vi "Shutdown.vi"(8 "error in":errorcluster, 11 "Serial Master in":refnum<class "Serial Master.lvclass">) -> (0 "error out":errorcluster)   [LabVIEW 2021, in "Serial Master.lvclass"]
doc: "This provides an interface for the master to close a connection to the slave."
uses:
  Serial Master.lvclass
  D:/my_projects/projects/Algorithms/Labview/21/Modbus_v121c/Network Protocol/Network Master/Network Master.lvclass
  Network Master.lvclass/Network Master.ctl
  Transmission Data Unit/Transmission Data Unit.lvclass
  Network Master.lvclass
  Serial Master.lvclass/Serial Master.ctl
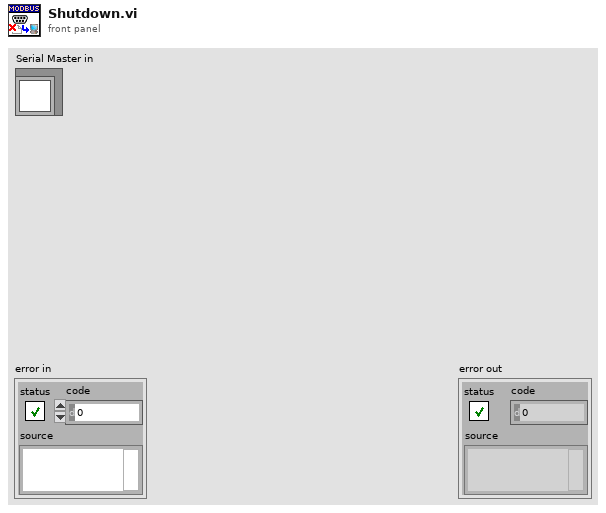
[diagram p1: front panel]
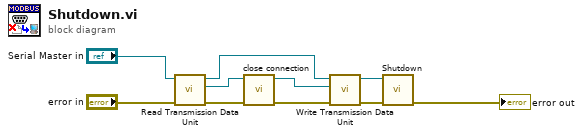
[diagram p0: block diagram]
diagram:
  n1 = call "Read Transmission Data Unit.vi"("error in (no error)"="error in", "Network Master in"="Serial Master in") -> ("error out"=w3:errorcluster, "Transmission Data Unit"=w4:refnum<class "Transmission Data Unit.lvclass">, "Network Master out"=w7:refnum<class "Serial Master.lvclass">)  [unwired: 7 in]
  n2 = call-dynamic "close connection.vi"("error in"=w3, "transmission data unit in"=w4) -> ("error out"=w1:errorcluster, "transmission data unit out"=w2:refnum<class "Transmission Data Unit.lvclass">)  [unwired: 8 in]
  n3 = call "Write Transmission Data Unit.vi"("error in (no error)"=w1, "Transmission Data Unit"=w2, "Network Master in"=w7) -> ("error out"=w6:errorcluster, "Network Master out"=w5:refnum<class "Serial Master.lvclass">)  [unwired: 7 in]
  n4 = call-parent "Shutdown.vi"("error in"=w6, "Network Master in"=w5) -> ("error out"=→"error out":errorcluster)  [unwired: 9 in]
